vi "Substitute Actor.vi"(10 "Substitute Actor in":refnum<class "Actor.lvclass">, 11 "Current Process State":refnum<class "Process State.lvclass">) -> (0 "error out":errorcluster, 2 "Substitute Actor out":refnum<class "Actor.lvclass">)   [LabVIEW 2025, in "Process States.lvlib" / "Process State.lvclass"]
doc: "(<B>Filename</B>: Actor Framework.lvlib:Actor.lvclass:Substitute Actor.vi)\n\nThis method copies information from the <b>Current Actor</b> to the <b>Substitute Actor</b>, including the to-self and the to-caller queue references. The purpose of this function is to allow an actor to define a method that replaces itself with another actor, useful for implementing a State Pattern Actor. Child classes should override this method to copy any additional fields that they need from the current to the substitute.\n\nThis method may return error code 678010: Illegal substitution. Overrides of this method may choose to return this error if the new actor is not one that is an appropriate substitute for the current actor, for whatever standards of \"appropriate\" are chosen for the current actor."
uses:
  Process State.lvclass
  <vilib>/ActorFramework/Actor/Actor.lvclass
  Process State.lvclass/Process State.ctl
  <vilib>/ni/Actors/State Actor/State Actor/State Actor.lvclass
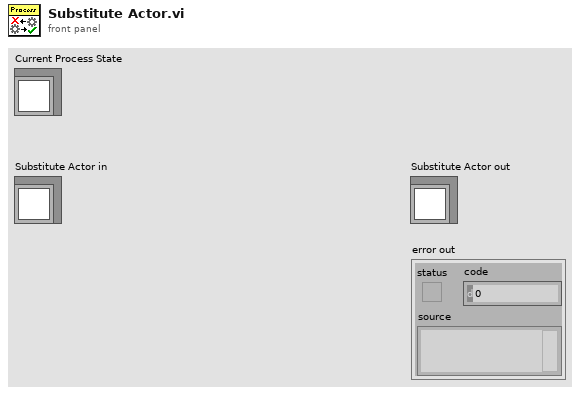
[diagram p1: front panel]
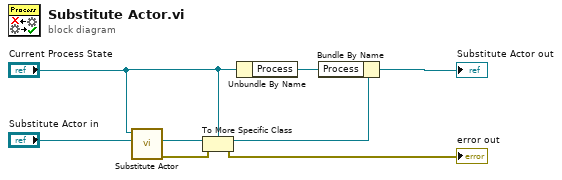
[diagram p0: block diagram]
diagram:
  n1 = call-parent "Substitute Actor.vi"("Substitute Actor in"="Substitute Actor in", "Current Actor"="Current Process State") -> ("error out"=w3:errorcluster, "Substitute Actor out"=w8:refnum<class "Actor.lvclass">)  [unwired: 8 in]
  n2 = To More Specific Class(target class="Current Process State", reference=w8, error in=w3) -> (specific class reference=w6:refnum<class "Process State.lvclass">, error out=→"error out":errorcluster)
  n3 = Unbundle By Name("Current Process State") -> ("Process"=w1:refnum<class "Message Enqueuer.lvclass">)
  n4 = Bundle By Name(cluster=w6, "Process"=w1) -> (→"Substitute Actor out":refnum<class "Process State.lvclass">)
